vi "Get Big&Small UPH.vi"(8 "error in (no error)":errorcluster, 10 "Model":string, 11 "Cluster":T2) -> (0 "error out":errorcluster, 3 "UPH":i16)   [LabVIEW 2014]
uses:
  Type'def/FTT Display Type.ctl
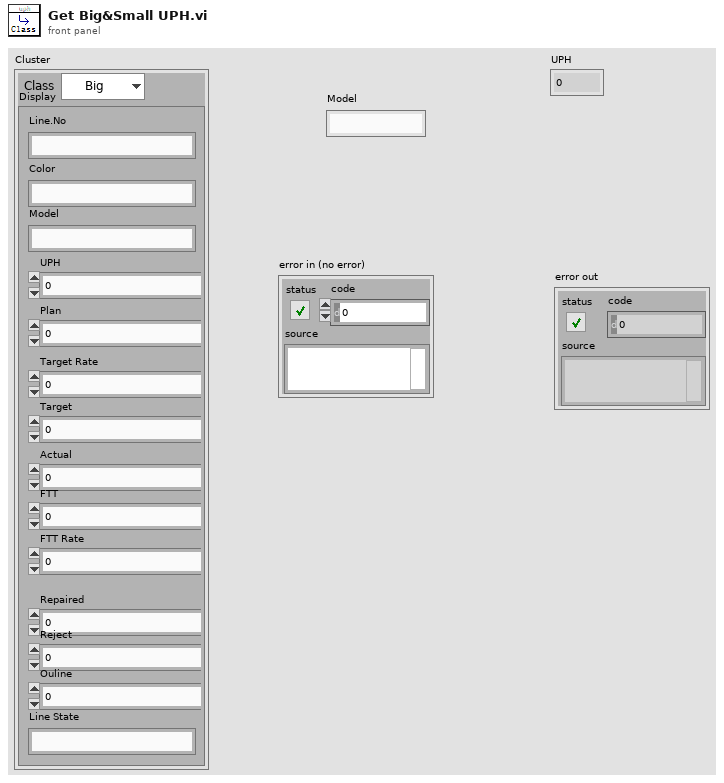
[diagram p1: front panel]
types:
  T1 = typedef "FTT Display Type.ctl" = cluster{"Line.No":string, "Model":string, "Color":string, "UPH":dbl, "Plan":dbl, "Target Rate":dbl, "Target ":dbl, "Actual":dbl, "FTT":dbl, "FTT Rate":dbl, "Repaired":dbl, "Reject":dbl, "Ouline":dbl, "Line State":string}
  T2 = cluster{"Display":T1, "Class":enum16{"Big", "Small"}}
  T3 = typedef "UPH Config.ctl" = cluster{"Line_No":string, "Model":string, "B_UPH ":i16, "S_UPH  ":i16, "Class":enum16{"Big", "Small"}}
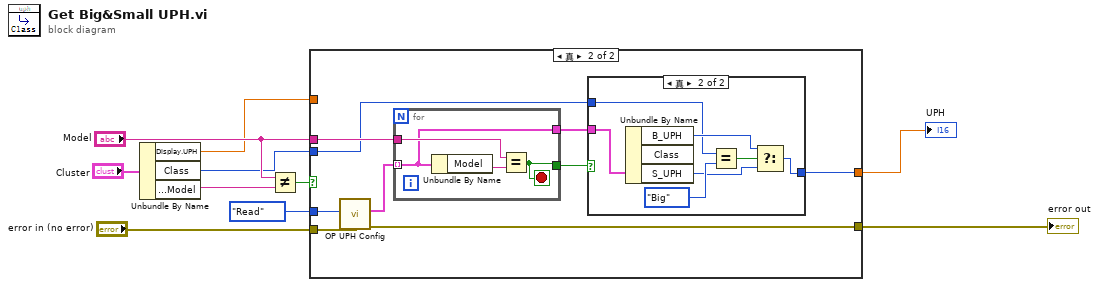
[diagram p0: block diagram]
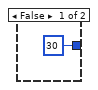
[diagram p3: hidden frame]
diagram:
  n1 = Unbundle By Name("Cluster") -> ("Display.UPH"=w2:dbl, "Class"=w1:enum16{"Big", "Small"}, "Display.Model"=w9:string)
  n2 = Not Equal?(x="Model", y=w9) -> (x != y?=w8:bool)
  n3 = case shown="真" w8 {
    tunnel: "error in (no error)" -> [w12 w21]
    tunnel: enum16{"init", "Read", "Write"}."Read" ("Enum") -> [_ w20]
    tunnel: w2 -> [w11 _]
    tunnel: "Model" -> [_ w18]
    tunnel: [w12 w17] -> w4
    tunnel: [w11 w14] -> w3
    tunnel: w1 -> [_ w13]
    frame False {
    }
    frame True {
      n4 = call "OP UPH Config.vi"("error in (no error)"=w21, "Enum"=w20) -> ("error out"=w17:errorcluster, "UPH out"=w19:T3[])  [unwired: 7 in, 1 out]
      n5 = for {
        tunnel: w19 -> [w31] mode=indexing
        tunnel: w18 -> [w32]
        tunnel: [w31] -> w15
        tunnel: [w30] -> w16
        stop <- w30 stop-if-true
        n6 = Unbundle By Name(w31) -> ("Model"=w33:string)
        n7 = Equal?(x=w32, y=w33) -> (x = y?=w30:bool)
      }
      n8 = case shown="真" w16 {
        tunnel: w15 -> [_ w29]
        tunnel: [i16 30 ("S_UPH") w24] -> w14
        tunnel: w13 -> [_ w23]
        frame False {
        }
        frame True {
          n9 = Unbundle By Name(w29) -> ("B_UPH"=w26:i16, "S_UPH"=w25:i16)  [unwired: 1 out]
          n10 = Equal?(x=w23, y=enum16{"Big", "Small"}."Big" ("Class")) -> (x = y?=w27:bool)
          n11 = Select(t=w26, s=w27, f=w25) -> (s? t:f=w24:i16)
        }
      }
    }
  }
  "error out" <- w4
  "UPH" <- w3
